vi "Home Single.vi"(8 "error in":errorcluster, 10 "Axis":enum16{"X", "Y", "Z", "U"}(ring), 11 "Gantry in":refnum<class "Gantry.lvclass">) -> (0 "error out":errorcluster, 3 "Gantry out":refnum<class "Gantry.lvclass">)   [LabVIEW 2026, in "Gantry.lvclass"]
uses:
  Gantry.lvclass
  Gantry.lvclass/Gantry.ctl
  Vec3d Class/Vec3d.lvclass
  <instrlib>/Aerotech Automation1/Aerotech Automation1.lvlib
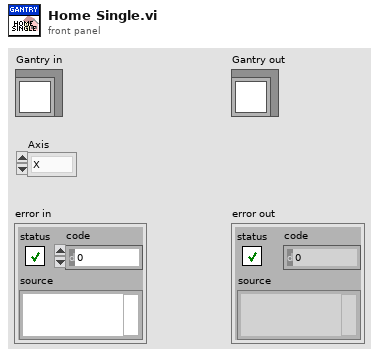
[diagram p1: front panel]
types:
  T1 = typedef "Virtual Modes.ctl" = enum16{"Nonvirtual", "Virtual"}
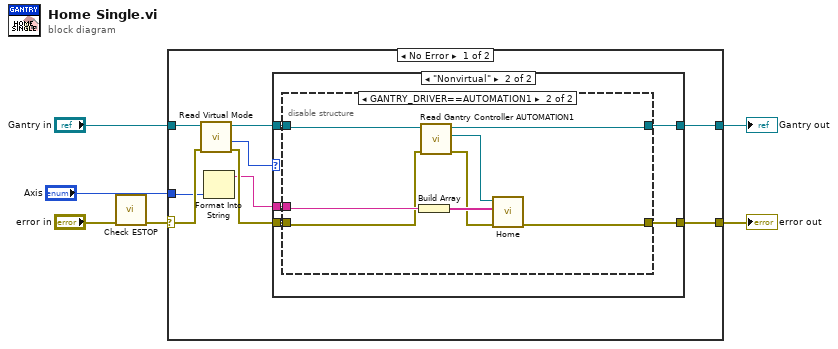
[diagram p0: block diagram]
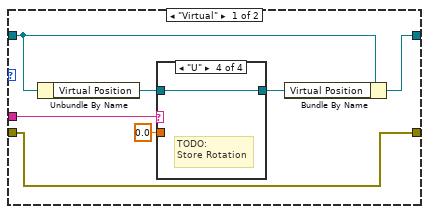
[diagram p2: hidden frame]
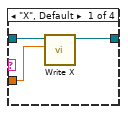
[diagram p3: hidden frame]
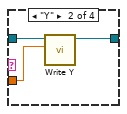
[diagram p4: hidden frame]
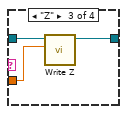
[diagram p5: hidden frame]
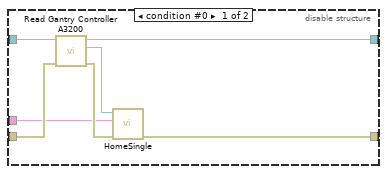
[diagram p6: hidden frame]
diagram:
  n1 = call "Check ESTOP.vi"("error in"="error in") -> ("error out"=w3:errorcluster)  [unwired: 10 in]
  n2 = case shown="No Error" w3 {
    selector: w3 -> [w10 w54]
    tunnel: [w15 w54] -> w6
    tunnel: [w14 w53] -> w5
    tunnel: "Gantry in" -> [w13 w53]
    tunnel: "Axis" -> [w8 _]
    frame No Error {
      n3 = call-dynamic "Read Virtual Mode.vi"("error in (no error)"=w10, "Gantry in"=w13) -> ("error out"=w9:errorcluster, "Virtual Mode"=w11:T1, "Gantry out"=w12:refnum<class "Gantry.lvclass">)  [unwired: 6 in, 1 out]
      n4 = Format Into String(w8) -> (resulting string=w7:string)  [unwired: 3 in, 1 out]
      n5 = case shown="\"Nonvirtual\"" w11 {
        tunnel: w12 -> [w20 w36]
        tunnel: w9 -> [w17 w35]
        tunnel: [w17 w37] -> w15
        tunnel: [w18 w34] -> w14
        tunnel: w7 -> [w16 w33]
        frame "Virtual" {
          n6 = Unbundle By Name(w20) -> ("Virtual Position"=w21:refnum<class "Vec3d.lvclass">)
          n7 = case shown="\"U\"" w16 {
            tunnel: 0.0 -> [w23 w26 w31 _]
            tunnel: w21 -> [w25 w28 w30 w32]
            tunnel: [w24 w27 w29 w32] -> w19
            frame "X", Default {
              n8 = call-dynamic "Write X.vi"("X"=w23, "Vec3d Class in"=w25) -> ("Vec3d Class out"=w24:refnum<class "Vec3d.lvclass">)  [unwired: 8 in, 1 out]
            }
            frame "Y" {
              n9 = call-dynamic "Write Y.vi"("Y"=w26, "Vec3d Class in"=w28) -> ("Vec3d Class out"=w27:refnum<class "Vec3d.lvclass">)  [unwired: 8 in, 1 out]
            }
            frame "Z" {
              n10 = call-dynamic "Write Z.vi"("Z"=w31, "Vec3d Class in"=w30) -> ("Vec3d Class out"=w29:refnum<class "Vec3d.lvclass">)  [unwired: 8 in, 1 out]
            }
            frame "U" {
              # "TODO: \nStore Rotation"
            }
          }
          n11 = Bundle By Name(cluster=w20, "Virtual Position"=w19) -> (w18:refnum<class "Gantry.lvclass">)
        }
        frame "Nonvirtual" {
          n12 = disable-structure shown="GANTRY_DRIVER==AUTOMATION1" {
            disable-tunnel: [w44 w45] -> w37
            disable-tunnel: w36 -> [w43 w49]
            disable-tunnel: w35 -> [w42 w46]
            disable-tunnel: [w39 w48] -> w34
            disable-tunnel: w33 -> [w38 w47]
            frame condition #0 {
              n13 = call "Read Gantry Controller A3200.vi"("error in (no error)"=w42, "Gantry in"=w43) -> ("error out"=w41:errorcluster, "A3200 controller out"=w40:refnum<k24>, "Gantry out"=w39:refnum<class "Gantry.lvclass">)  [unwired: 7 in]
              n14 = call "HomeSingle.vi"("error in (no error)"=w41, "axis name"=w38, "controller in"=w40) -> ("error out"=w44:errorcluster)  [unwired: 7 in, 1 out]
            }
            frame condition #1 (active) {
              n15 = Build Array(w47) -> (w51:string[])
              n16 = call "Read Gantry Controller AUTOMATION1.vi"("error in (no error)"=w46, "Gantry in"=w49) -> ("error out"=w50:errorcluster, "Controller AUTOMATION1"=w52:refnum<k24>, "Gantry out"=w48:refnum<class "Gantry.lvclass">)  [unwired: 7 in]
              n17 = call <instrlib>:"Home.vi"("error in (no error)"=w50, "axes"=w51, "Controller Refnum"=w52) -> ("error out"=w45:errorcluster)  [unwired: 7 in, 1 out]
            }
          }
        }
      }
    }
    frame Error {
    }
  }
  "error out" <- w6
  "Gantry out" <- w5
